vi "DFD Chebyshev Design.vi"(4 "passband ripple [dB]":dbl=1.0 format="%.2f", 6 "fs [Hz]":dbl=1.0 format="%.2f", 7 "filter type":T1(ring), 8 "error in (no error)":errorcluster, 9 "low cutoff freq [Hz]":dbl=0.12, 10 "high cutoff freq [Hz]":dbl=0.45, 11 "order":i32=2) -> (0 "error out":errorcluster, 3 "filter out":T2={"mSRate_Fs"=1.0, "mSRate_Version"="2.0", "mSRate_Comments"="", "mSRate_OrgCoef"={"type"=enum."Undefined", "gain"=1.0, "coef a (k)"=[], "coef b (v)"=[]}, "mSRate_CurCoef"={"type"=enum."Undefined", "gain"=1.0, "coef a (k)"=[], "coef b (v)"=[]}, "mSRate_Quantized?"=FALSE, "mSRate_QCoef"={"type"=enum."Undefined", "gain"=1.0, "coef a (k)"=[], "coef b (v)"=[]}, "mSRate_QSettings"=[], "mSRate_Order"=0, "mSRate_Scaling"={"mSRate_ScaleByPowerOf2?"=FALSE, "mSRate_ScaleType"=enum."No Norm"}} {"mSRate_QSettings"."source" items=["Coef a/k"=0, "Coef b/v"=7, "Input"=1, "Output"=2, "Multiplicand"=3, "Product"=4, "Sum"=5, "Delay"=6, "Gain"=8]})   [LabVIEW 2017, in "NI_DigFilterLicensed.lvlib"]
doc: "Creates a digital Chebyshev infinite impulse response (IIR) filter."
uses:
  <vilib>/addons/Digital Filter Design/NI_DigFilterLicensed.lvlib
  <vilib>/addons/Digital Filter Design/_Objects.llb/DFD Filter Obj.ctl
  <vilib>/addons/Digital Filter Design/_Objects.llb/DFD Filter Coef.ctl
  <vilib>/addons/Digital Filter Design/_Objects.llb/DFD Filter Structure Type Selector.ctl
  <vilib>/addons/Digital Filter Design/_Objects.llb/dfd_Internal Quantization Settings.ctl
  <vilib>/addons/Digital Filter Design/_Objects.llb/dfd_Internal Quantization Srcs.ctl
  <vilib>/addons/Digital Filter Design/_Objects.llb/DFD Coef Norm Type.ctl
  <vilib>/addons/Digital Filter Design/NI_DigFilter_Design.lvlib
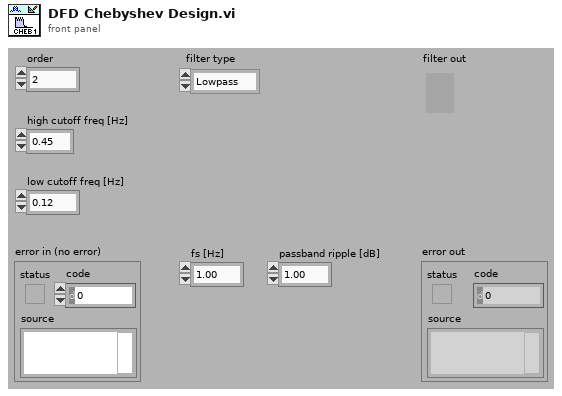
[diagram p1: front panel]
types:
  T1 = enum16{"Lowpass", "Highpass", "Bandpass", "Bandstop"}
  T2 = typedef "NI_DigFilterLicensed.lvlib/DFD Filter Obj.ctl" = cluster{"mSRate_Fs":dbl, "mSRate_Version":string, "mSRate_Comments":string, "mSRate_OrgCoef":T3, "mSRate_CurCoef":T3, "mSRate_Quantized?":bool, "mSRate_QCoef":T3, "mSRate_QSettings":T5[], "mSRate_Order":i32, "mSRate_Scaling":cluster{"mSRate_ScaleByPowerOf2?":bool, "mSRate_ScaleType":T7}}
  T3 = typedef "NI_DigFilterLicensed.lvlib/DFD Filter Coef.ctl" = cluster{"type":T4, "gain":dbl, "coef a (k)":dbl[], "coef b (v)":dbl[]}
  T4 = typedef "NI_DigFilterLicensed.lvlib/DFD Filter Structure Type Selector.ctl" = enum16{"Undefined", "FIR Direct Form", "FIR Direct Form Transposed", "FIR Symmetric", "FIR Antisymmetric", "IIR Direct Form I", "IIR Direct Form I Transposed", "IIR Direct Form II", "IIR Direct Form II Transposed", "IIR Cascaded Second Order Sections Form I", "IIR Cascaded Second Order Sections Form I Transposed", "IIR Cascaded Second Order Sections Form II", "IIR Cascaded Second Order Sections Form II Transposed", "Lattice Allpass (basic sections)", "Lattice Allpass (one multiplier sections)", "Lattice Allpass (normalized sections)", "Lattice AR (basic sections)", "Lattice AR (one multiplier sections)", "Lattice AR (normalized sections)", "Lattice MA (minimum phase)", "Lattice MA (maximum phase)", "Lattice ARMA (basic sections)", "Lattice ARMA (one multiplier sections)", "Lattice ARMA (normalized sections)"}
  T5 = typedef "NI_DigFilterLicensed.lvlib/dfd_Internal Quantization Settings.ctl" = cluster{"source":T6, "wl":i16, "iwl":i16, "overflow mode":enum16{"Saturation", "Wrap"}, "rounding mode":enum16{"Nearest", "Truncation"}, "signed?":bool}
  T6 = typedef "NI_DigFilterLicensed.lvlib/dfd_Internal Quantization Srcs.ctl" = u16
  T7 = typedef "NI_DigFilterLicensed.lvlib/DFD Coef Norm Type.ctl" = enum16{"No Norm", "Time Domain 1-Norm", "Time Domain 2-Norm", "Time Domain Inf-Norm"}
  T8 = enum16{"Butterworth", "Chebyshev", "Inv Chebyshev", "Elliptic", "Bessel"}
  T9 = cluster{"passband ripple [dB]":dbl, "passband ripple [dB]":dbl}
  T10 = typedef "NI_DigFilterLicensed.lvlib/DFD Pole-Zero.ctl" = cluster{"value":cdb, "z attr":cluster{"real":bool, "lp":bool, "uc":bool}, "order":i32}
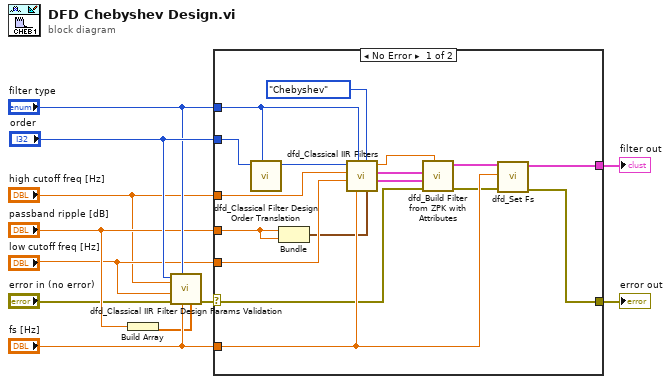
[diagram p0: block diagram]
diagram:
  n1 = Build Array("passband ripple [dB]") -> (w2:dbl[])
  n2 = call <vilib>:"dfd_Classical IIR Filter Design Params Validation.vi"("params"=w2, "fs [Hz]"="fs [Hz]", "filter type"="filter type", "error in (no error)"="error in (no error)", "low cutoff freq: fl"="low cutoff freq [Hz]", "high cutoff freq: fh"="high cutoff freq [Hz]", "order"="order") -> ("error out"=w1:errorcluster)  [unwired: 4 out]
  n3 = case shown="No Error" w1 {
    selector: w1 -> [w16 w29]
    tunnel: [w13 w29] -> w11
    tunnel: [w14 _] -> w10
    tunnel: "order" -> [w28 _]
    tunnel: "filter type" -> [w27 _]
    tunnel: "passband ripple [dB]" -> [w26 _]
    tunnel: "low cutoff freq [Hz]" -> [w25 _]
    tunnel: "high cutoff freq [Hz]" -> [w24 _]
    tunnel: "fs [Hz]" -> [w23 _]
    frame No Error {
      n4 = call <vilib>:"dfd_Classical Filter Design Order Translation.vi"("filter type"=w27, "input order"=w28) -> ("order for design"=w19:i32)  [unwired: 9 out]
      n5 = Bundle("passband ripple [dB]"=w26, "passband ripple [dB]"=w26) -> (w12:T9)  [unwired: 1 out]
      n6 = call <vilib>:"dfd_Classical IIR Filters.vi"("ripples [dB]"=w12, "filter design"=T8."Chebyshev", "fs [Hz]"=w23, "filter type"=w27, "low cutoff freq: fl"=w25, "high cutoff freq: fh"=w24, "order"=w19) -> ("poles"=w20:T10[], "zeros"=w21:T10[], "gain"=w22:dbl)  [unwired: 1 in, 1 out]
      n7 = call <vilib>:"dfd_Build Filter from ZPK with Attributes.vi"("gain"=w22, "error in (no error)"=w16, "poles"=w20, "zeros"=w21) -> ("error out"=w18:errorcluster, "filter out"=w17:T2)  [unwired: 6 out]
      n8 = call <vilib>:"dfd_Set Fs.vi"("error in (no error)"=w18, "fs [Hz]"=w23, "filter in"=w17) -> ("error out"=w13:errorcluster, "filter out"=w14:T2)  [unwired: 7 out]
    }
    frame Error {
    }
  }
  "filter out" <- w10
  "error out" <- w11
